vi "Get Channel Configuration.vi"(8 "error in (no error)":errorcluster, 10 "Channel":T2, 11 "EPU452 in":refnum<class "EPU452.lvclass">) -> (0 "error out":errorcluster, 1 "Channel Config":T1=enum."Disabled", 2 "Response":string, 3 "EPU452 out":refnum<class "EPU452.lvclass">)   [LabVIEW 2018, in "EPU452.lvclass"]
uses:
  EPU452.lvclass
  Controls/Channels.ctl
  Controls/Channel Config.ctl
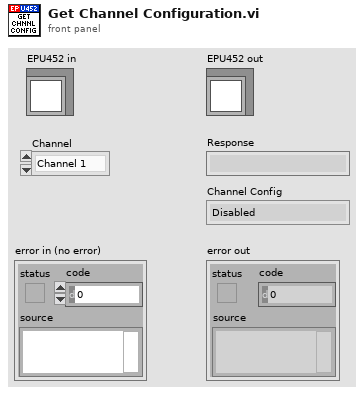
[diagram p1: front panel]
types:
  T1 = typedef "EPU452.lvclass/Channel Config.ctl" = enum16{"Unknown", "Disabled", "Voltmeter", "pH/ISE", "Pt 1k RTD", "10 k Thermistor", "dO2", "Biosensor", "Conductivity"}
  T2 = typedef "EPU452.lvclass/Channels.ctl" = enum16{"Channel 1", "Channel 2", "Channel 3", "Channel 4"}
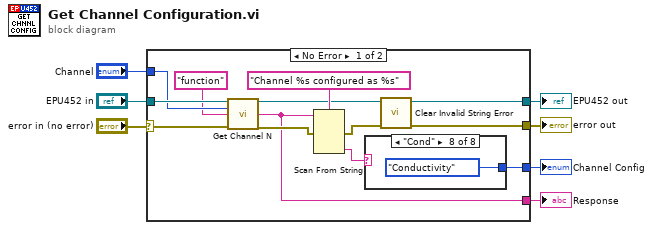
[diagram p0: block diagram]
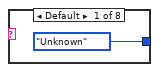
[diagram p2: hidden frame]
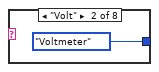
[diagram p3: hidden frame]
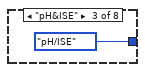
[diagram p4: hidden frame]
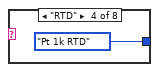
[diagram p5: hidden frame]
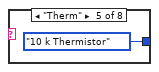
[diagram p6: hidden frame]
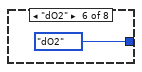
[diagram p7: hidden frame]
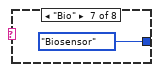
[diagram p8: hidden frame]
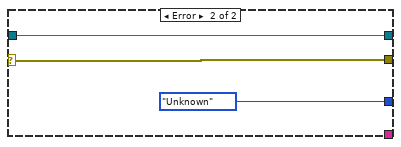
[diagram p9: hidden frame]
diagram:
  n1 = case shown="No Error" "error in (no error)" {
    selector: "error in (no error)" -> [w19 w31]
    tunnel: [w10 w31] -> w6
    tunnel: [w11 w30] -> w4
    tunnel: "EPU452 in" -> [w20 w30]
    tunnel: "Channel" -> [w18 _]
    tunnel: [w9 Channel_Config."Unknown" ("Channel Config")] -> w2
    tunnel: [w8 _] -> w1
    frame No Error {
      n2 = call "Get Channel N.vi"("EPU452 in"=w20, "Channel"=w18, "Function"="function", "error in (no error)"=w19) -> ("EPU452 out"=w13:refnum<class "EPU452.lvclass">, "Response"=w8:string, "error out"=w15:errorcluster)  [unwired: 9 in]
      n3 = Scan From String(format string="Channel %s configured as %s", input string=w8, error in=w15) -> (error out=w14:errorcluster, output 2=w12:string)  [unwired: 4 in, 2 out]
      n4 = case shown="\"Cond\"" w12 {
        tunnel: [Channel_Config."Unknown" ("Channel Config") Channel_Config."Voltmeter" ("Channel Config") Channel_Config."pH/ISE" ("Channel Config") Channel_Config."Pt 1k RTD" ("Channel Config") Channel_Config."10 k Thermistor" ("Channel Config") Channel_Config."dO2" ("Channel Config") Channel_Config."Biosensor" ("Channel Config") Channel_Config."Conductivity" ("Channel Config")] -> w9
        frame Default {
        }
        frame "Volt" {
        }
        frame "pH&ISE" {
        }
        frame "RTD" {
        }
        frame "Therm" {
        }
        frame "dO2" {
        }
        frame "Bio" {
        }
        frame "Cond" {
        }
      }
      n5 = call "Clear Invalid String Error.vi"("error in (no error)"=w14, "EPU452 in"=w13) -> ("error out"=w10:errorcluster, "EPU452 out"=w11:refnum<class "EPU452.lvclass">)  [unwired: 8 in]
    }
    frame Error {
    }
  }
  "error out" <- w6
  "EPU452 out" <- w4
  "Channel Config" <- w2
  "Response" <- w1
